vi "InstrParam.vi"(4 "queue out":refnum<queue>, 6 "user event out":refnum<user-event>, 8 "error in (no error)":errorcluster caption="entrée d'erreur (pas d'erreur)", 10 "InstrParam":string, 11 "SR400 en entrée":refnum<class "LSCI332.lvclass"> caption="DNL_LabVIEW Object in") -> (0 "error out":errorcluster caption="sortie d'erreur", 3 "SR400 en sortie":refnum<class "LSCI332.lvclass"> caption="DNL_LabVIEW Object out")   [LabVIEW 2019, in "LSCI332.lvclass"]
uses:
  LSCI332.lvclass
  C:/Programmes Labview/LabScanV1A/DevicesClass/BaseDevice/BaseDevice.lvclass
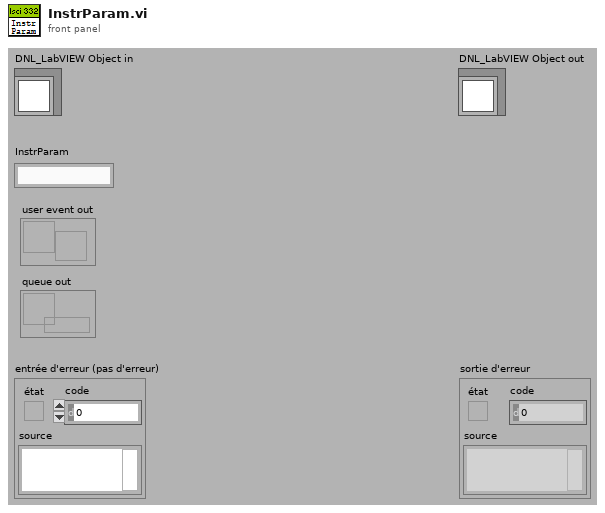
[diagram p1: front panel]
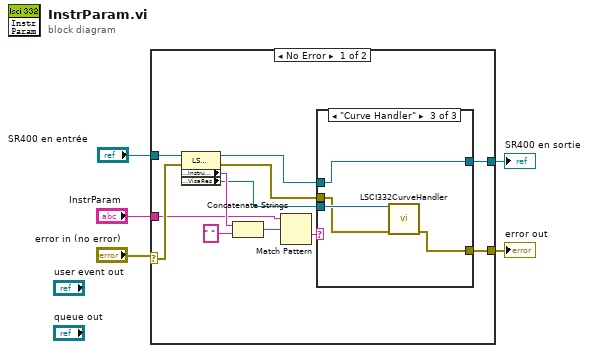
[diagram p0: block diagram]
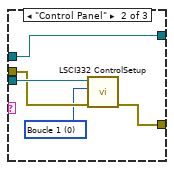
[diagram p3: hidden frame]
diagram:
  n1 = case shown="No Error" "error in (no error)" {
    selector: "error in (no error)" -> [w16 w29]
    tunnel: "SR400 en entrée" -> [w17 w30]
    tunnel: [w12 w30] -> w3
    tunnel: [w9 w29] -> w2
    tunnel: "InstrParam" -> [w6 _]
    frame No Error {
      n2 = property class="LSCI332.lvclass"(reference=w17, error in=w16) -> (reference out=w11:refnum<class "LSCI332.lvclass">, error out=w10:errorcluster, "Accessor:InstrumentName"=w14:string, "Accessor:VisaRes"=w8:refnum<visa-resource-name>)
      n3 = Concatenate Strings(w14, " " ("chaîne")) -> (w7:string)
      n4 = Match Pattern(string=w6, regular expression=w7) -> (after substring=w13:string)  [unwired: 1 in, 3 out]
      n5 = case shown="\"Curve Handler\"" w13 {
        tunnel: [w19 w24 w28] -> w12
        tunnel: w11 -> [w19 w24 w28]
        tunnel: w10 -> [w18 w22 w26]
        tunnel: [w18 w21 w25] -> w9
        tunnel: w8 -> [_ w23 w27]
        frame Default {
        }
        frame "Control Panel" {
          w20 = u32 0 items=["Boucle 1", "Boucle 2"] ("Boucle(1)")
          n6 = call <userlib>:"LSCI332 ControlSetup.vi"("error in"=w22, "Boucle(1)"=w20, "VISA Rsrc"=w23) -> ("error out"=w21:errorcluster)  [unwired: 6 in]
        }
        frame "Curve Handler" {
          n7 = call <userlib>:"LSCI332CurveHandler.vi"("VISA Rsrc"=w27, "error in"=w26) -> ("error out"=w25:errorcluster)  [unwired: 13 in]
        }
      }
    }
    frame Error {
    }
  }
  "error out" <- w2
  "SR400 en sortie" <- w3
